vi "Algo_Selector_UI_string_to_enum.vi"(8 "error in (no error)":errorcluster, 11 "Algo Type":string) -> (0 "error out":errorcluster, 3 "Algo type":T1(ring))   [LabVIEW 2014]
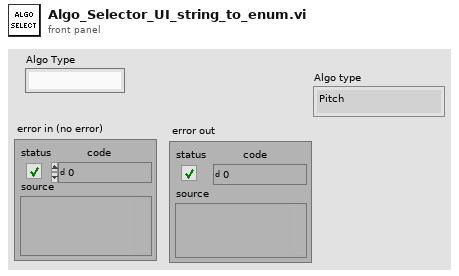
[diagram p1: front panel]
types:
  T1 = enum16{"Pitch", "Circlular_Dia", "LipGap", "Angle", "BarbHeight", "Linear", "Projected Distance_Type_1", " Projected Distance_Type_2", "Projected Distance_Type_3", "AET Max", "AET Min", "TT_Width", "Lancing", "WND", "Linear_Lenght1", "Linear_Lenght2", "Side_E", "Side_E1", "Top_E"}
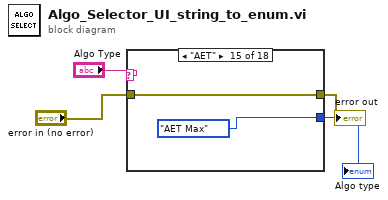
[diagram p0: block diagram]
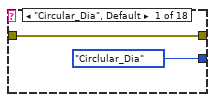
[diagram p2: hidden frame]
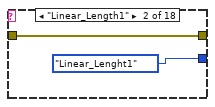
[diagram p3: hidden frame]
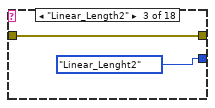
[diagram p4: hidden frame]
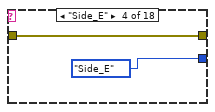
[diagram p5: hidden frame]
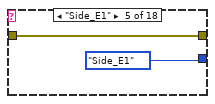
[diagram p6: hidden frame]
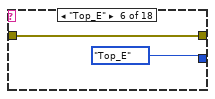
[diagram p7: hidden frame]
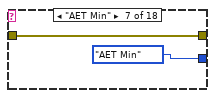
[diagram p8: hidden frame]
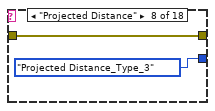
[diagram p9: hidden frame]
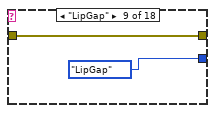
[diagram p10: hidden frame]
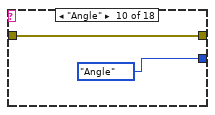
[diagram p11: hidden frame]
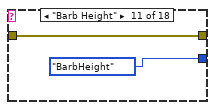
[diagram p12: hidden frame]
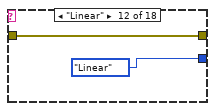
[diagram p13: hidden frame]
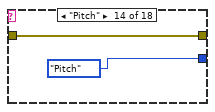
[diagram p15: hidden frame]
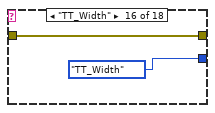
[diagram p16: hidden frame]
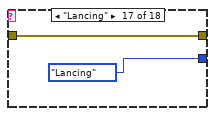
[diagram p17: hidden frame]
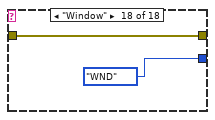
[diagram p18: hidden frame]
diagram:
  n1 = case shown="\"AET\"" "Algo Type" {
    tunnel: "error in (no error)" -> [w6 w8 w10 w12 w14 w16 w18 w20 w22 w24 w26 w28 w29 w31 w33 w35 w37 w39]
    tunnel: [w6 w8 w10 w12 w14 w16 w18 w20 w22 w24 w26 w28 w29 w31 w33 w35 w37 w39] -> w2
    tunnel: [T1."Circlular_Dia" ("Algo type") T1."Linear_Lenght1" ("Algo type") T1."Linear_Lenght2" ("Algo type") T1."Side_E" ("Algo type") T1."Side_E1" ("Algo type") T1."Top_E" ("Algo type") T1."AET Min" ("Algo type") T1."Projected Distance_Type_3" ("Algo type") T1."LipGap" ("Algo type") T1."Angle" ("Algo type") T1."BarbHeight" ("Algo type") T1."Linear" ("Algo type") _ T1."Pitch" ("Algo type") T1."AET Max" ("Algo type") T1."TT_Width" ("Algo type") T1."Lancing" ("Algo type") T1."WND" ("Algo type")] -> w1
    frame "Circular_Dia", Default {
    }
    frame "Linear_Length1" {
    }
    frame "Linear_Length2" {
    }
    frame "Side_E" {
    }
    frame "Side_E1" {
    }
    frame "Top_E" {
    }
    frame "AET Min" {
    }
    frame "Projected Distance" {
    }
    frame "LipGap" {
    }
    frame "Angle" {
    }
    frame "Barb Height" {
    }
    frame "Linear" {
    }
    frame "Linear 2" {
    }
    frame "Pitch" {
    }
    frame "AET" {
    }
    frame "TT_Width" {
    }
    frame "Lancing" {
    }
    frame "Window" {
    }
  }
  "error out" <- w2
  "Algo type" <- w1
